vi "Magazine_Teleop.vi"(11 "Joystick_In":T1) -> ()   [LabVIEW 2019]
uses:
  Globals/Magazine_Globals.vi
  Subsystems/Magazine/Magazine_Cluster.ctl
  Utility_VIs/Joystick_Controls.ctl
panel:
  in  "Magazine_Speed":dbl
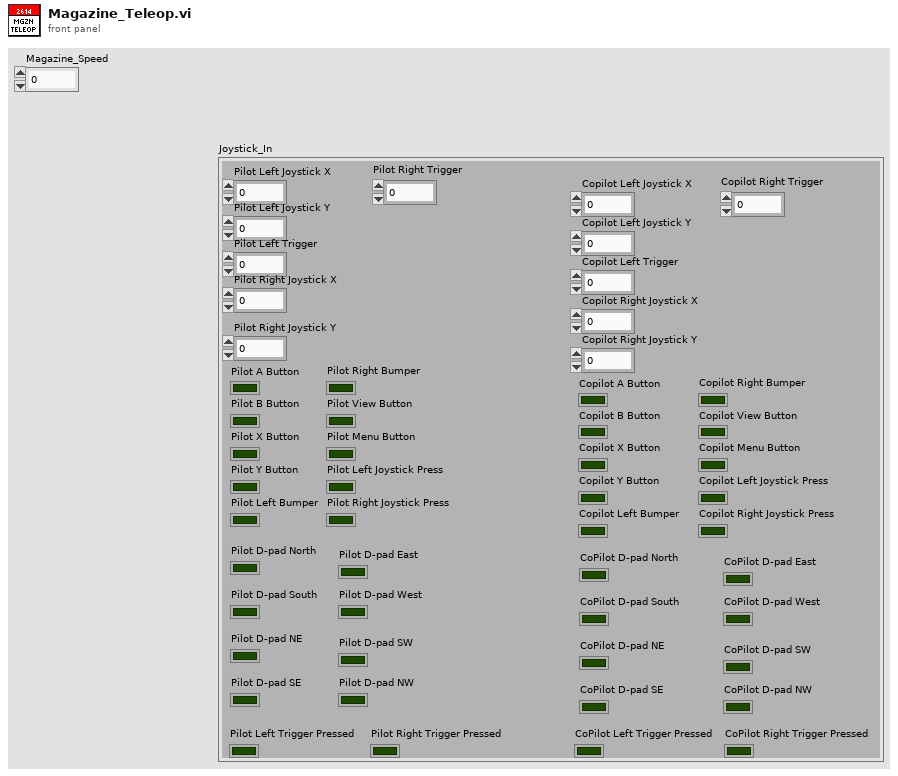
[diagram p1: front panel]
types:
  T1 = typedef "Joystick_Controls.ctl" = cluster{"Pilot Left Joystick X":dbl, "Pilot Left Joystick Y":dbl, "Pilot A Button":bool, "Pilot B Button":bool, "Pilot X Button":bool, "Pilot Y Button":bool, "Pilot Left Bumper":bool, "Pilot Right Bumper":bool, "Pilot View Button":bool, "Pilot Menu Button":bool, "Pilot Left Joystick Press":bool, "Pilot Right Joystick Press":bool, "Pilot Left Trigger":dbl, "Pilot Right Joystick X":dbl, "Pilot Right Joystick Y":dbl, "Pilot Right Trigger":dbl, "Copilot Left Joystick X":dbl, "Copilot Left Joystick Y":dbl, "Copilot A Button":bool, "Copilot B Button":bool, "Copilot X Button":bool, "Copilot Y Button":bool, "Copilot Left Bumper":bool, "Copilot Right Bumper":bool, "Copilot View Button":bool, "Copilot Menu Button":bool, "Copilot Left Joystick Press":bool, "Copilot Right Joystick Press":bool, "Copilot Left Trigger":dbl, "Copilot Right Joystick X":dbl, "Copilot Right Joystick Y":dbl, "Copilot Right Trigger":dbl, "Pilot D-pad North":bool, "Pilot D-pad South":bool, "Pilot D-pad East":bool, "Pilot D-pad West":bool, "Pilot D-pad NE ":bool, "Pilot D-pad SE":bool, "Pilot D-pad SW":bool, "Pilot D-pad NW":bool, "CoPilot D-pad North":bool, "CoPilot D-pad South":bool, "CoPilot D-pad East":bool, "CoPilot D-pad West":bool, "CoPilot D-pad NE":bool, "CoPilot D-pad SE":bool, "CoPilot D-pad SW":bool, "CoPilot D-pad NW":bool, "Pilot Left Trigger Pressed":bool, "Pilot Right Trigger Pressed":bool, "CoPilot Left Trigger Pressed":bool, "CoPilot Right Trigger Pressed":bool}
  T2 = typedef "Magazine_Cluster.ctl" = cluster{"Control_States":enum16{"No-Op", "Loading", "Fire", "Unjam", "Manual"}, "Fire":bool, "Magazine_Throttle":dbl}
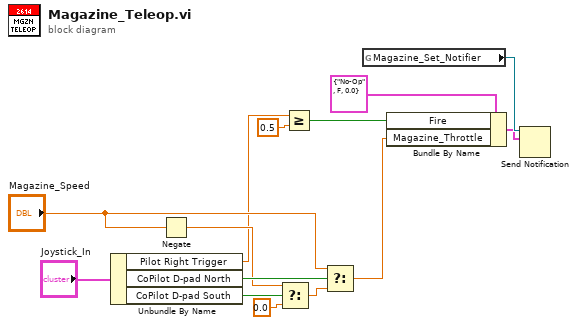
[diagram p0: block diagram]
diagram:
  n1 = Unbundle By Name("Joystick_In") -> ("Pilot Right Trigger"=w4:dbl, "CoPilot D-pad North"=w10:bool, "CoPilot D-pad South"=w9:bool)
  n2 = Negate(x="Magazine_Speed") -> (-x=w5:dbl)
  n3 = Select(t=w5, s=w9, f=0.0) -> (s? t:f=w8:dbl)
  n4 = Greater Or Equal?(x=w4, y=0.5) -> (x >= y?=w2:bool)
  n5 = Select(t="Magazine_Speed", s=w10, f=w8) -> (s? t:f=w1:dbl)
  n6 = global read "Magazine_Globals.vi" "Magazine_Set_Notifier"() -> (w13:refnum<notifier>)
  n7 = Bundle By Name(cluster=T2 {"Control_States"=enum."No-Op", "Fire"=FALSE, "Magazine_Throttle"=0.0} ("Magazine_Cluster"), "Fire"=w2, "Magazine_Throttle"=w1) -> (w11:T2)
  n8 = Send Notification(notification=w11, notifier=w13) -> ()  [unwired: 1 in, 2 out]
